vi "Public Get Context.vi"(8 "error in (no error)":errorcluster, 11 "Mock Process in":refnum<class "Mock Process.lvclass">) -> (0 "error out":errorcluster, 2 "Context":refnum<class "Process.lvclass">, 3 "Mock Process out":refnum<class "Mock Process.lvclass">)   [LabVIEW 2020, in "Mock Process.lvclass"]
uses:
  Mock Process.lvclass
  C:/git/astemes-triarc-framework/source/Framework/Process/Process.lvclass
  Framework/Process/Process.lvclass
  Framework/Process/Process.lvclass/Process.ctl
  Framework/Process/Public/Lifecycle/Get Lifecycle State.vi
  <vilib>/Utility/error.llb/Clear Errors.vi
  <vilib>/Utility/error.llb/Error Cluster From Error Code.vi
  Mock Process.lvclass/Mock Process.ctl
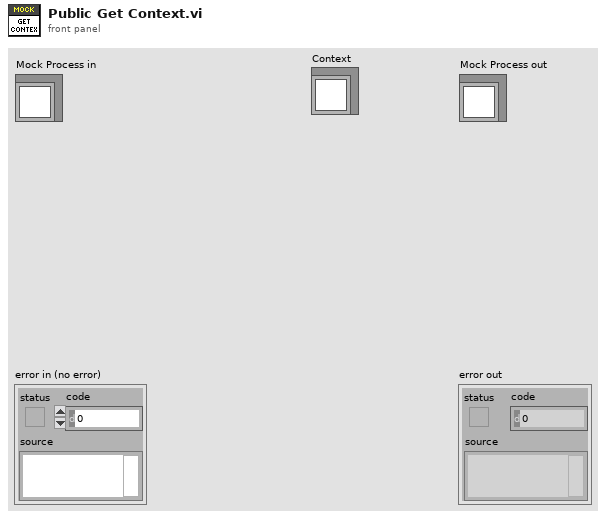
[diagram p1: front panel]
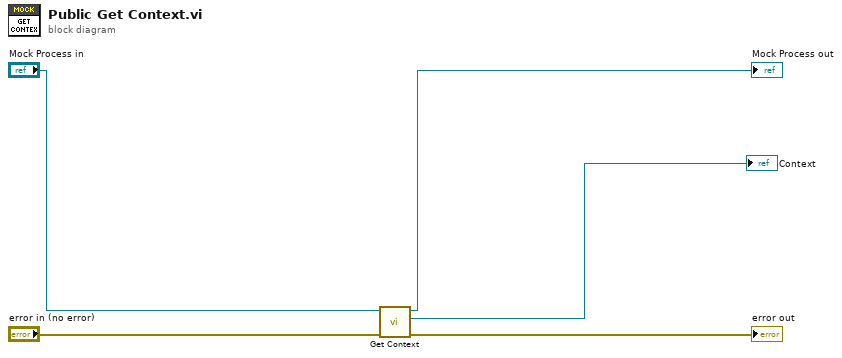
[diagram p0: block diagram]
diagram:
  n1 = call "Get Context.vi"("error in (no error)"="error in (no error)", "Process In"="Mock Process in") -> ("error out"=→"error out":errorcluster, "Context"=→"Context":refnum<class "Process.lvclass">, "Process Out"=→"Mock Process out":refnum<class "Mock Process.lvclass">)  [unwired: 6 in, 1 out]
